vi "Get Cell Cost.vi"(8 "error in (no error)":errorcluster, 9 "y":i32, 10 "x":i32, 11 "map reference in":refnum<data-value>) -> (0 "error out":errorcluster, 1 "found?":bool, 2 "cost":dbl, 3 "map reference out":refnum<data-value>)   [LabVIEW 2017, in "NI_Robotics_OccupancyGridWorldMap.lvclass"]
doc: "Returns the cost of entering the cell in the occupancy grid map at the <B>x</B>- and <B>y</B>-coordinates you specify."
uses:
  <vilib>/robotics/Navigation/shared/WorldMap/OccupancyGridWorldMap/NI_Robotics_OccupancyGridWorldMap.lvclass
  <vilib>/robotics/Navigation/shared/MapNode/OccupancyGridNode/NI_Robotics_OccupancyGridMapNode.lvclass
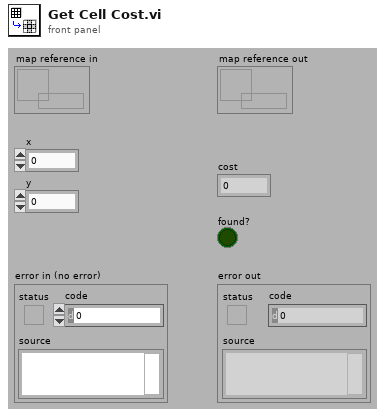
[diagram p1: front panel]
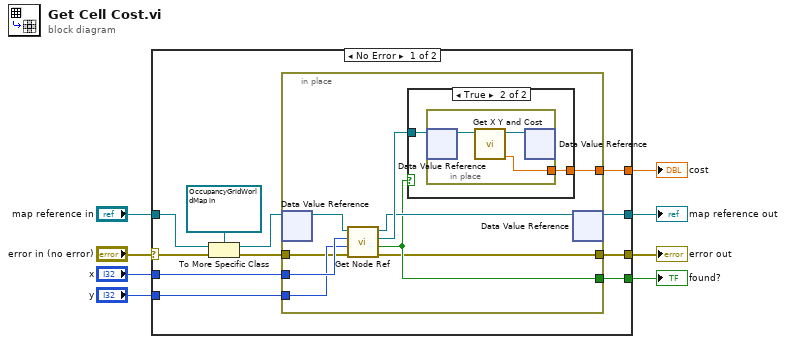
[diagram p0: block diagram]
diagram:
  n1 = case shown="No Error" "error in (no error)" {
    selector: "error in (no error)" -> [w13 w35]
    tunnel: [w19 w34] -> w4
    tunnel: [w14 w35] -> w3
    tunnel: "x" -> [w18 _]
    tunnel: "y" -> [w17 _]
    tunnel: [w16 _] -> w6
    tunnel: [w15 _] -> w5
    tunnel: "map reference in" -> [w11 w34]
    frame No Error {
      n2 = To More Specific Class(target class=refnum<data-value> refnum ("World Map Reference"), reference=w11, error in=w13) -> (specific class reference=w9:refnum<data-value>, error out=w12:errorcluster)
      n3 = in-place {
        in-place-border: w18 -> [w27]
        in-place-border: w17 -> [w26]
        in-place-border: w12 -> [w25]
        in-place-border: [w22] -> w16
        in-place-border: [w21] -> w15
        in-place-border: [w20] -> w14
        n4 = in-place-dvr #1(w9) -> (w28:refnum<class "NI_Robotics_OccupancyGridWorldMap.lvclass">)  [unwired: 1 out]
        n5 = call <vilib>:"Get Node Ref.vi"("error in (no error)"=w25, "y"=w26, "x"=w27, "OccupancyGridWorldMap in"=w28) -> ("error out"=w20:errorcluster, "Found"=w21:bool, "element"=w24:refnum<data-value>, "OccupancyGridWorldMap out"=w23:refnum<class "NI_Robotics_OccupancyGridWorldMap.lvclass">)  [unwired: 4 in]
        n6 = case shown="True" w21 {
          tunnel: w24 -> [_ w30]
          tunnel: [_ w29] -> w22
          frame False {
          }
          frame True {
            n7 = in-place {
              in-place-border: [w31] -> w29
              n8 = in-place-dvr #2(w30) -> (w33:refnum<class "NI_Robotics_OccupancyGridMapNode.lvclass">)  [unwired: 1 out]
              n9 = call-dynamic "Get X Y and Cost.vi"("OccupancyGridMapNode in"=w33) -> ("Cost"=w31:dbl, "OccupancyGridMapNode out"=w32:refnum<class "NI_Robotics_OccupancyGridMapNode.lvclass">)  [unwired: 7 in, 2 out]
              n10 = in-place-dvr #2(w32) -> ()  [unwired: 2 out]
            }
          }
        }
        n11 = in-place-dvr #1(w23) -> (w19:refnum<data-value>)  [unwired: 1 out]
      }
    }
    frame Error {
    }
  }
  "error out" <- w3
  "map reference out" <- w4
  "cost" <- w6
  "found?" <- w5
